vi "Launch Valves.vi"(8 "error in (no error)":errorcluster, 11 "Storage Line in":refnum<class "Storage Line.lvclass">) -> (0 "error out":errorcluster, 3 "Storage Line out":refnum<class "Storage Line.lvclass">)   [LabVIEW 2015, in "cRIO-Carbondioxide.lvlib" / "CO2-Actor.lvlib" / "Storage Line.lvclass"]
uses:
  Storage Line.lvclass
  Valve/Action.ctl
  <vilib>/ActorFramework/Actor/Actor.lvclass
  Storage Line.lvclass/Storage Line.ctl
  CO2 Actor/CO2 Actor.lvclass
  Valve/Valve.lvclass
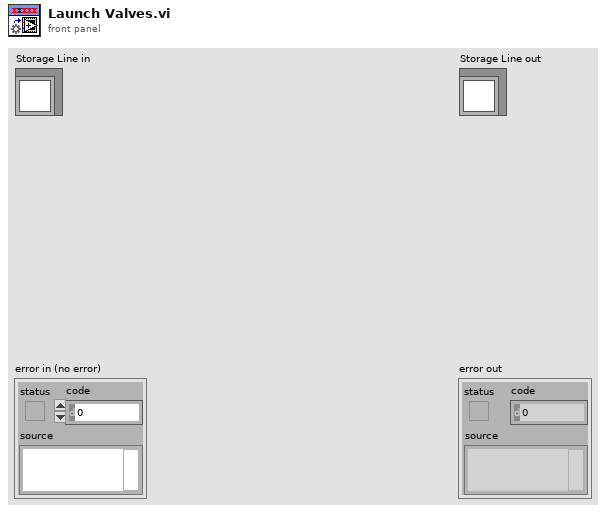
[diagram p1: front panel]
types:
  T1 = typedef "Action.ctl" = enum16{"Open", "Close", "None"}
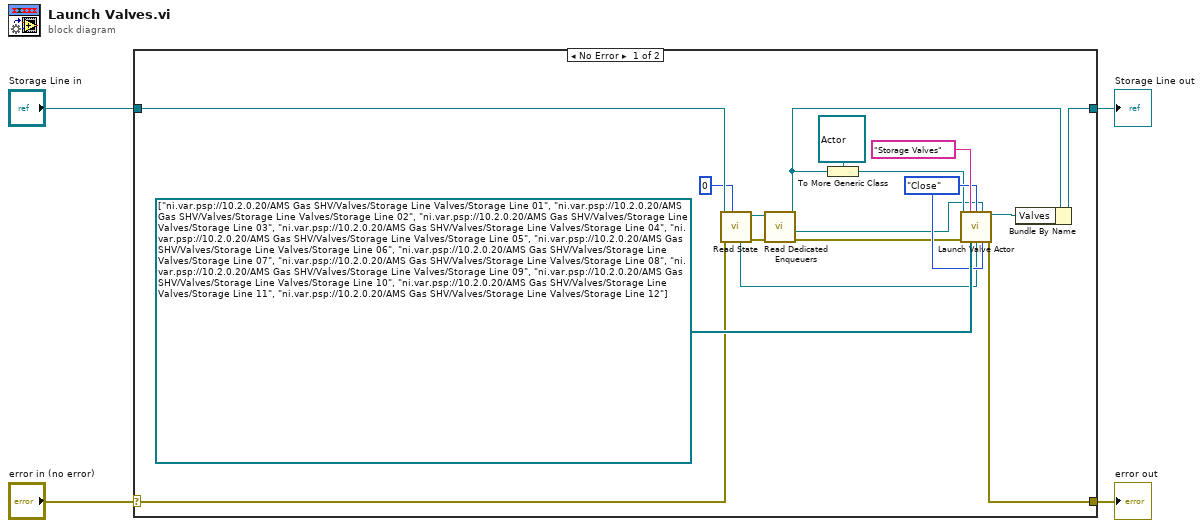
[diagram p0: block diagram]
diagram:
  n1 = case shown="No Error" "error in (no error)" {
    selector: "error in (no error)" -> [w8 w23]
    tunnel: [w21 w23] -> w3
    tunnel: [w17 w22] -> w1
    tunnel: "Storage Line in" -> [w10 w22]
    frame No Error {
      w18 = Action."Close" ("Start Action (Open)")
      n2 = call "Read State.vi"("timeout in ms (-1)"=0, "error in (no error)"=w8, "Storage Line in"=w10) -> ("error out"=w7:errorcluster, "Storage Line out"=w9:refnum<class "Storage Line.lvclass">, "Line StateQ"=w6:refnum<queue>)  [unwired: 4 in, 2 out]
      n3 = call "Read Dedicated Enqueuers.vi"("error in (no error)"=w7, "CO2 Actor in"=w9) -> ("error out"=w13:errorcluster, "DedicatedEnQrs"=w11:refnum<queue>, "CO2 Actor out"=w12:refnum<class "Storage Line.lvclass">)  [unwired: 6 in, 1 out]
      n4 = To More Generic Class(target class=refnum<class "Actor.lvclass"> refnum ("Caller Actor in"), reference=w12) -> (generic class reference=w15:refnum<class "Actor.lvclass">)
      n5 = call "Launch Valve Actor.vi"("Caller Actor in"=w15, "Name"="Storage Valves", "Start Action (Open)"=w18, "DedicatedEnQrs"=w11, "error in (no error)"=w13, "SHV"=refnum<k21>[] ["ni.var.psp://10.2.0.20/AMS Gas SHV/Valves/Storage Line Valves/Storage Line 01", "ni.var.psp://10.2.0.20/AMS Gas SHV/Valves/Storage Line Valves/Storage Line 02", "ni.var.psp://10.2.0.20/AMS Gas SHV/Valves/Storage Line Valves/Storage Line 03", "ni.var.psp://10.2.0.20/AMS Gas SHV/Valves/Storage Line Valves/Storage Line 04", "ni.var.psp://10.2.0.20/AMS Gas SHV/Valves/Storage Line Valves/Storage Line 05", "ni.var.psp://10.2.0.20/AMS Gas SHV/Valves/Storage Line Valves/Storage Line 06", "ni.var.psp://10.2.0.20/AMS Gas SHV/Valves/Storage Line Valves/Storage Line 07", "ni.var.psp://10.2.0.20/AMS Gas SHV/Valves/Storage Line Valves/Storage Line 08", "ni.var.psp://10.2.0.20/AMS Gas SHV/Valves/Storage Line Valves/Storage Line 09", "ni.var.psp://10.2.0.20/AMS Gas SHV/Valves/Storage Line Valves/Storage Line 10", "ni.var.psp://10.2.0.20/AMS Gas SHV/Valves/Storage Line Valves/Storage Line 11", "ni.var.psp://10.2.0.20/AMS Gas SHV/Valves/Storage Line Valves/Storage Line 12"], "StateQ"=w6, "Stop Action (Close)"=w18) -> ("Caller-To-Actor Enqueuer"=w16:refnum<class "Message Enqueuer.lvclass">, "error out"=w21:errorcluster)  [unwired: 6 in]
      n6 = Bundle By Name(cluster=w12, "Valves"=w16) -> (w17:refnum<class "Storage Line.lvclass">)
    }
    frame Error {
    }
  }
  "error out" <- w3
  "Storage Line out" <- w1
